vi "init.vi"(8 "error in (no error)":errorcluster, 11 "dummyCam in":refnum<class "dummyCam.lvclass">) -> (0 "error out":errorcluster, 3 "dummyCam out":refnum<class "dummyCam.lvclass">)   [LabVIEW 2018, in "dummyCam.lvclass"]
uses:
  dummyCam.lvclass
  _cameraBase/_cameraBase.lvclass
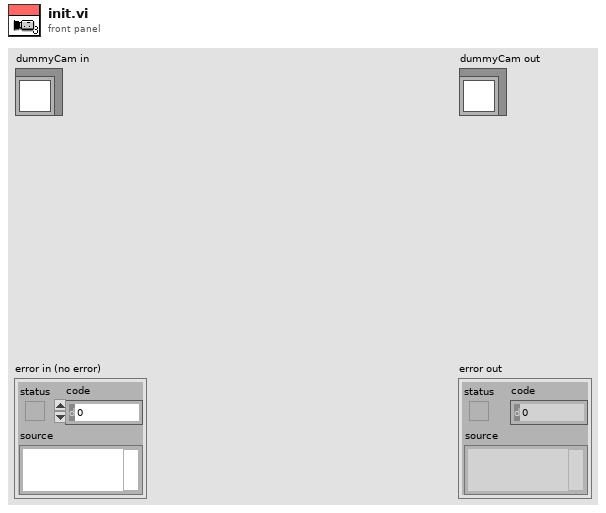
[diagram p1: front panel]
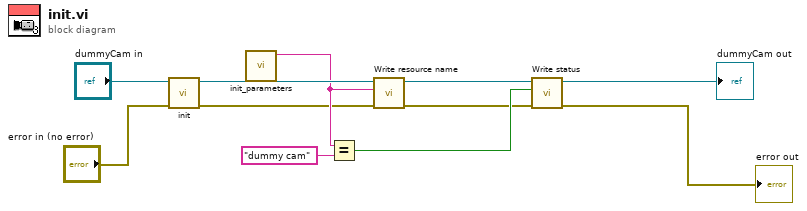
[diagram p0: block diagram]
diagram:
  n1 = call-parent "init.vi"("error in (no error)"="error in (no error)", "_cameraBase in"="dummyCam in") -> ("error out"=w1:errorcluster, "_cameraBase out"=w9:refnum<class "dummyCam.lvclass">)  [unwired: 8 in]
  n2 = call "init_parameters.vi"() -> ("Resource name out"=w8:string)  [unwired: 10 in]
  n3 = Equal?(x=w8, y="dummy cam") -> (x = y?=w4:bool)
  n4 = call-dynamic "Write resource name.vi"("error in (no error)"=w1, "resource name"=w8, "_cameraBase in"=w9) -> ("error out"=w2:errorcluster, "_cameraBase out"=w6:refnum<class "dummyCam.lvclass">)  [unwired: 7 in]
  n5 = call-dynamic "Write status.vi"("error in (no error)"=w2, "status"=w4, "_cameraBase in"=w6) -> ("error out"=→"error out":errorcluster, "_cameraBase out"=→"dummyCam out":refnum<class "dummyCam.lvclass">)  [unwired: 7 in]
